vi "Get Events.vi"(11 "Sensor View in":refnum<class "Sensor View.lvclass">) -> (2 "Events":T1, 3 "Sensor View out":refnum<class "Sensor View.lvclass">)   [LabVIEW 2013, in "Sensor View.lvlib" / "Sensor View.lvclass"]
uses:
  Sensor View.lvclass
  Typedef/Events.ctl
  Sensor View.lvclass/Sensor View.ctl
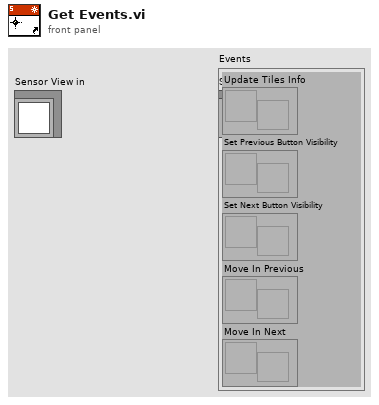
[diagram p1: front panel]
types:
  T1 = typedef "Sensor View.lvlib/Sensor View.lvclass/Events.ctl" = cluster{"Update Tiles Info":refnum<user-event>, "Set Previous Button Visibility":refnum<user-event>, "Set Next Button Visibility":refnum<user-event>, "Move In Previous":refnum<user-event>, "Move In Next":refnum<user-event>}
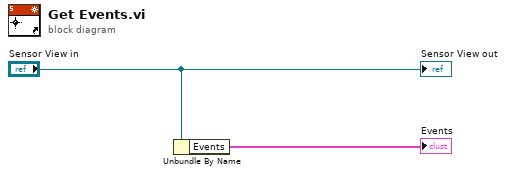
[diagram p0: block diagram]
diagram:
  n1 = Unbundle By Name("Sensor View in") -> ("Events"=→"Events":T1)
  "Sensor View out" <- "Sensor View in"
